vi "参数.vi"() -> ()   [LabVIEW 2012]
uses:
  <vilib>/vision/Image Controls.llb/IMAQ Image.ctl
panel:
  out "本次任务":T1
  in  "当前状态":T2(ring)
  in  "全局关机":bool
  in  "ErrorLog":string
  out "运行参数":T4
  # "错误代码\n0 示波器初始化错误\n1 Cam1初始化错误\n2 能量功率表头初始化错误\n\n\n12 能量功率表头测量错误"
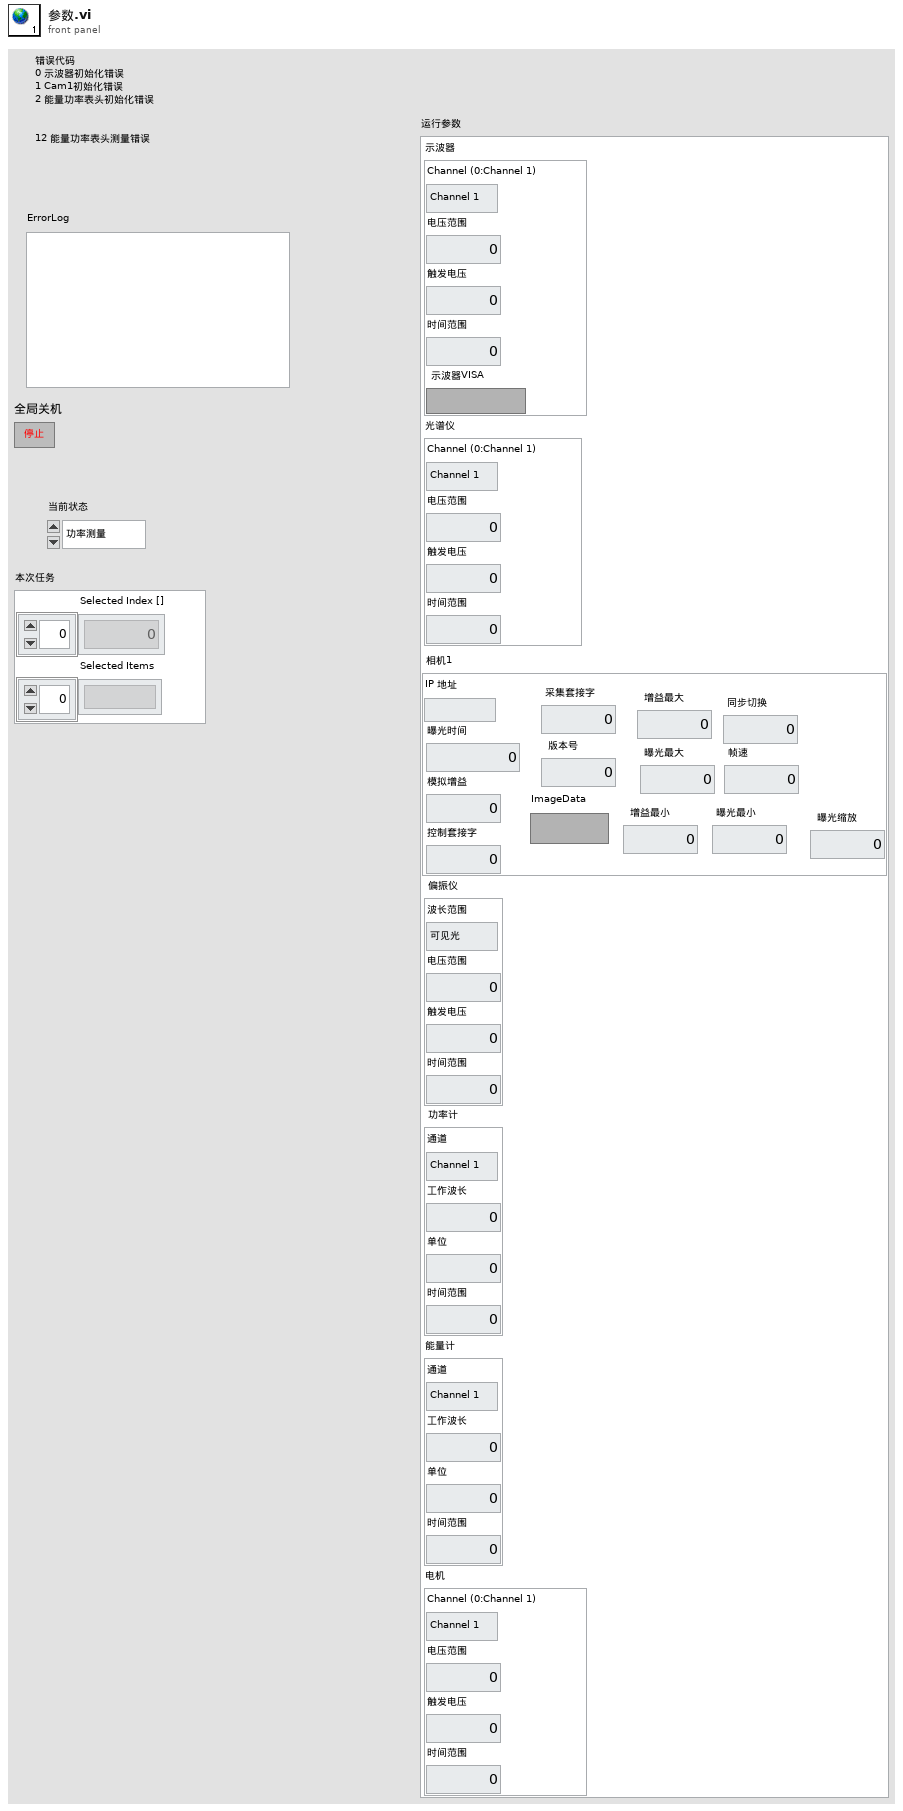
[diagram p1: front panel]
types:
  T1 = cluster{"Selected Index []":i32[], "Selected Items":string[]}
  T2 = enum16{"功率测量", "能量测量", "光谱测量", "时间波形", "近远场", "偏振"}
  T3 = typedef "IMAQ Image.ctl" = refnum<image>
  T4 = cluster{"示波器":cluster{"Channel (0:Channel 1)":enum16{"Channel 1", "Channel 2", "Channel 3", "Channel 4"}, "电压范围":dbl, "触发电压":dbl, "时间范围":dbl, " 示波器VISA":refnum<visa-resource-name>}, "光谱仪":cluster{"Channel (0:Channel 1)":enum16{"Channel 1", "Channel 2", "Channel 3", "Channel 4"}, "电压范围":u64, "触发电压":u64, "时间范围":u64}, " 相机1":cluster{"曝光时间":i32, "模拟增益":i32, "控制套接字":i32, "IP 地址":string, " 采集套接字":i32, "  版本号":i32, "ImageData":T3, "  增益最大":i32, "  增益最小":i32, " 曝光最大":i32, " 曝光最小":i32, " 帧速":i32, " 同步切换":i32, "  曝光缩放":i32}, " 偏振仪":cluster{"波长范围":enum16{"可见光", "近红外"}, "电压范围":u64, "触发电压":u64, "时间范围":u64}, " 功率计":cluster{"通道":enum16{"Channel 1", "Channel 2"}, "工作波长":u64, "单位":u64, "时间范围":u64}, "能量计":cluster{"通道":enum16{"Channel 1", "Channel 2"}, "工作波长":u64, "单位":u64, "时间范围":u64}, "电机":cluster{"Channel (0:Channel 1)":enum16{"Channel 1", "Channel 2", "Channel 3", "Channel 4"}, "电压范围":u64, "触发电压":u64, "时间范围":u64}}
diagram:
